vi "Request Compatible Hardware.vi"(8 "error in (no error)":errorcluster, 11 "Server UI in":refnum<class "Server UI.lvclass">) -> (0 "error out":errorcluster, 3 "Server UI out":refnum<class "Server UI.lvclass">)   [LabVIEW 2017, in "Server UI.lvlib" / "Server UI.lvclass"]
uses:
  Server UI.lvclass
  \\Mac\Home/Documents/MAL-Framework/user.lib/Common Components/Msmt UI/Measurement UI.lvclass
  C:/Program Files (x86)/National Instruments/LabVIEW 2017/vi.lib/ActorFramework/Actor/Actor.lvclass
  Server UI.lvclass/Server UI.ctl
  MAL-Framework/user.lib/Common Components/Msmt UI/Measurement UI.lvclass/Measurement UI.ctl
  <vilib>/ActorFramework/Actor/Actor.lvclass/Actor.ctl
  MAL-Framework/user.lib/Common Components/Controller/Messages/Find Compatible Hardware for Measurement Msg/Find Compatible Hardware for Measurement Msg.lvclass/Find Compatible Hardware for Measurement Msg.ctl
  <vilib>/ActorFramework/Message Enqueuer/Message Enqueuer.lvclass/Message Enqueuer.ctl
  Controller/Messages/Request Compatible Hardware from Client Msg/Request Compatible Hardware from Client Msg.lvclass/Request Compatible Hardware from Client Msg.ctl
  Read Connected Clients.vi
  MAL-Framework/user.lib/Common Components/Msmt UI/Accessors/Read Measurement.vi
  Read Connection Showing.vi
  <vilib>/ActorFramework/Message Enqueuer/Enqueue.vi
  MAL-Framework/user.lib/Common Components/Controller/Messages/Find Compatible Hardware for Measurement Msg/Find Compatible Hardware for Measurement Msg.lvclass
  C:/Program Files (x86)/National Instruments/LabVIEW 2017/vi.lib/ActorFramework/Message/Message.lvclass
  Controller/Messages/Request Compatible Hardware from Client Msg/Request Compatible Hardware from Client Msg.lvclass
  <vilib>/ActorFramework/Message Priority Queue/Priority Enqueue.vi
  <vilib>/ActorFramework/Actor/Actor.lvclass
  MAL-Framework/user.lib/Common Components/Msmt UI/Measurement UI.lvclass
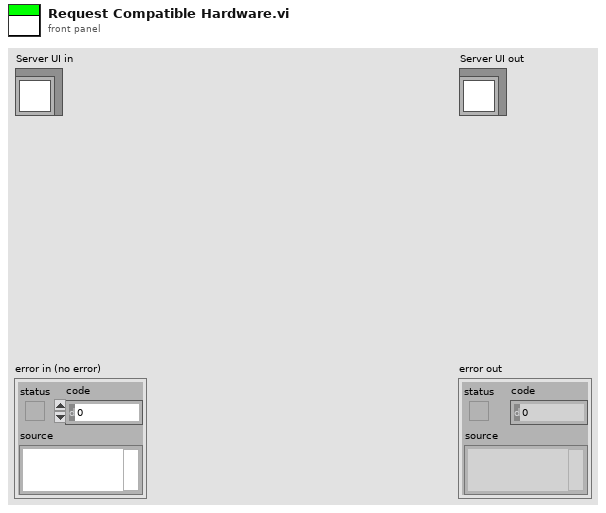
[diagram p1: front panel]
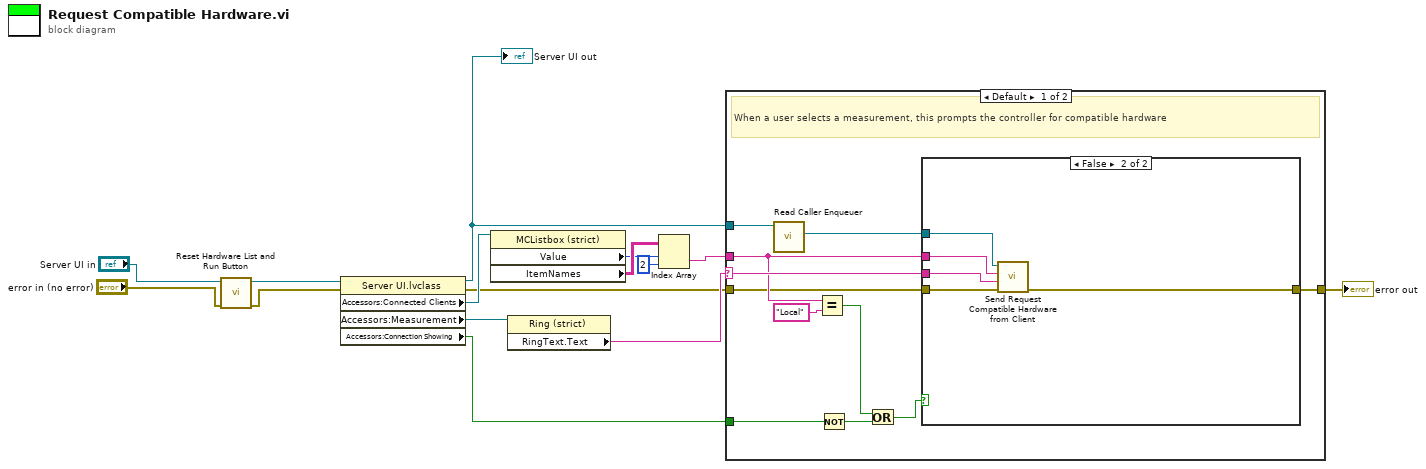
[diagram p0: block diagram]
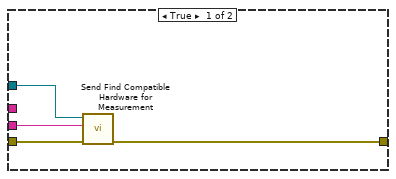
[diagram p2: hidden frame]
diagram:
  n1 = call "Reset Hardware List and Run Button.vi"("error in (no error)"="error in (no error)", "Measurement UI in"="Server UI in") -> ("error out"=w4:errorcluster, "Measurement UI out"=w2:refnum<class "Server UI.lvclass">)  [unwired: 8 in]
  n2 = property class="Server UI.lvclass"(reference=w2, error in=w4) -> (reference out=w10:refnum<class "Server UI.lvclass">, error out=w8:errorcluster, "Accessors:Connected Clients"=w15:refnum<vi>, "Accessors:Measurement"=w11:refnum<vi>, "Accessors:Connection Showing"=w6:bool)
  "Server UI out" <- w10
  n3 = property class="MCListbox (strict)"(reference=w15) -> ("Value"=w13:i32, "ItemNames"=w14:string[][])  [unwired: 1 in, 2 out]
  n4 = property class="Ring (strict)"(reference=w11) -> ("RingText.Text"=w12:string)  [unwired: 1 in, 2 out]
  n5 = Index Array(array=w14, index (row)=w13, index (col)=2 ("disabled index (col)")) -> (element=w9:string)
  n6 = case shown="Default" w12 {
    selector: w12 -> [w24 _]
    tunnel: w10 -> [w26 _]
    tunnel: w9 -> [w18 _]
    tunnel: w6 -> [w19 _]
    tunnel: w8 -> [w17 w36]
    tunnel: [w16 w36] -> w7
    frame Default {
      # "When a user selects a measurement, this prompts the controller for compatible hardware"
      n7 = call <vilib>:"Read Caller Enqueuer.vi"("Actor"=w26) -> ("Caller Enqueuer"=w25:refnum<class "Message Enqueuer.lvclass">)  [unwired: 10 in]
      n8 = Equal?(x=w18, y="Local") -> (x = y?=w22:bool)
      n9 = Not(x=w19) -> (.not. x?=w20:bool)
      n10 = Or(x=w22, y=w20) -> (x .or. y?=w21:bool)
      n11 = case shown="False" w21 {
        tunnel: w17 -> [w28 w35]
        tunnel: [w27 w34] -> w16
        tunnel: w25 -> [w29 w33]
        tunnel: w24 -> [w30 w32]
        tunnel: w18 -> [_ w31]
        frame True {
          n12 = call "Send Find Compatible Hardware for Measurement.vi"("error in (no error)"=w28, "Measurement Name"=w30, "Message Enqueuer"=w29) -> ("error out"=w27:errorcluster)  [unwired: 7 in, 1 out]
        }
        frame False {
          n13 = call "Send Request Compatible Hardware from Client.vi"("error in (no error)"=w35, "Measurement"=w32, "ConnectionID"=w31, "Message Enqueuer"=w33) -> ("error out"=w34:errorcluster)  [unwired: 6 in, 1 out]
        }
      }
    }
    frame "Select One:" {
    }
  }
  "error out" <- w7
